vi "Dashboard Main.vi"() -> ()   [LabVIEW 2019]
uses:
  Vision/Vision Mode.ctl
  <vilib>/Utility/miscctls.llb/LVRowAndColumnTypeDef.ctl
  <vilib>/event_ctls.llb/eventvkey.ctl
  <vilib>/Rock Robotics/Network Tables/NT Read Numeric Array.vi
  <vilib>/Rock Robotics/WPI/Dashboard/WPI_DashboardLogging Global.vi
  <vilib>/Rock Robotics/Network Tables/NT Read Boolean.vi
panel:
  in  "Camera Settings Right":T1={"Frame Rate"=30, "Compression"=30, "Size"=1, "DB Camera Config"=FALSE} {"Frame Rate" scale=1.0..30.0; "Compression" scale=100.0..-1.0; "Size" items=["640x480", "320x240", "160x120"]}
  in  "Camera Name Right":string(combo)="No Camera Selection"
  out "Camera Perf":string
  in  "Camera Settings":T1={"Frame Rate"=30, "Compression"=30, "Size"=1, "DB Camera Config"=FALSE} {"Frame Rate" scale=1.0..30.0; "Compression" scale=100.0..-1.0; "Size" items=["640x480", "320x240", "160x120"]}
  in  "TCP":refnum<k5>
  in  "Rec Mode":enum32{"Stop", "Record", "Playback"}(radio)
  out "Robot IP":string
  out "Image Message":string="Timeout in Camera Communications"
  in  "Dashboard Tab":T2(tab)
  in  "Select Auto":string(combo)="Select Autonomous ..."
  out "NT Connection":bool
  out "MotorChart R":cluster{"Numeric":dbl, "Numeric":dbl}(graph)
  out "MotorChart L":cluster{"Numeric":dbl, "Numeric":dbl}(graph)
  out "MotorSliders R":cluster{"MotorSlide1":dbl, "MotorSlide2":dbl} {"MotorSlide2" scale=-1.0..1.0 scale format="%#_2e"; "MotorSlide1" scale=-1.0..1.0 scale format="%#_2e"}
  out "MotorSliders L":cluster{"MotorSlide1":dbl, "MotorSlide2":dbl} {"MotorSlide2" scale=-1.0..1.0 scale format="%#_2e"; "MotorSlide1" scale=-1.0..1.0 scale format="%#_2e"}
  out "Gyro":dbl(knob) scale=0.0..360.0
  out "JS1 Z":dbl(slide) scale=-1.0..1.0 scale format="%#_2e"
  out "JS1 Graph":cluster{"X":dbl, "Y":dbl}[](graph)
  out "JS1 Buttons":T3
  out "JS2 Z":dbl(slide) scale=-1.0..1.0 scale format="%#_2e"
  out "JS2 Graph":cluster{"X":dbl, "Y":dbl}[](graph)
  out "JS2 Buttons":T3
  out "Mode":T4(ring)=enum."Auto Disabled"
  out "Right Camera Perf":cluster{"Bandwidth (Mbps)":dbl, "FPS":dbl}
  out "Camera Image Right":T5(plugin-control)
  in  "DB/String 9":string
  in  "DB/String 8":string
  in  "DB/String 7":string
  in  "DB/String 6":string
  in  "DB/String 5":string
  in  "DB/String 4":string
  in  "DB/String 3":string
  in  "DB/String 2":string
  in  "DB/String 1":string
  in  "DB/String 0":string
  in  "DB/Slider 0":dbl(slide) scale=0.0..5.0
  in  "DB/Slider 1":dbl(slide) scale=0.0..5.0
  in  "DB/Slider 2":dbl(slide) scale=0.0..5.0
  in  "DB/Slider 3":dbl(slide) scale=0.0..5.0
  out "DB/LED 3":bool
  out "DB/LED 2":bool
  out "DB/LED 1":bool
  out "DB/LED 0":bool
  in  "DB/Button 3":bool
  in  "DB/Button 2":bool
  in  "DB/Button 1":bool
  in  "DB/Button 0":bool caption="New Name"
  out "Width":i32
  out "Centroid.x":sgl
  in  "Centerpoint Target":dbl=160.0
  in  "PID gains":T6={"proportional gain (Kc)"=0.01, "integral time (Ti, min)"=0.0, "derivative time (Td, min)"=0.0} {"derivative time (Td, min)" format="%.3f"; "integral time (Ti, min)" format="%.3f"; "proportional gain (Kc)" format="%.3f"}
  in  "Vision Mode":T7
  out "Number of Matches":i32
  in  "Test Slider":dbl(slide) scale=0.0..100.0 scale format="%#_3g"
  in  "On/Off":bool caption="Solenoid"
  in  "Test Name":u16(ring) items=["Select the test to run..."]
  in  "Test Tree":string(tree)
  in  "Motor":cluster{"Value":dbl, "Enable":bool} {"Value" scale=-1.0..1.0 scale format="%#_3g"}
  out "Progress":T8 {"Test Progress" scale=0.0..100.0}
  in  "Rev/Fwd":cluster{"Forward":bool, "Reverse":bool}
  in  "Test Ring":u16(ring) items=["Monochrome", "Color"]
  out "Cmd Status":string
  in  "Execute Command":bool
  in  "Command Params":string[][](table)
  in  "Command Selection":i32(listbox)
  in  "CheckList":i32(listbox)
  out "Tree":string(tree)
  out "Camera Image":T5(plugin-control)
  out "Background":bool
  in  "Camera Name":string(combo)="No Camera Selection"
  # "HW"
  # "HW"
  # "Joysticks"
  # "Drive Motors"
  # "Front"
  # "Right"
  # "Left"
  # "Back"
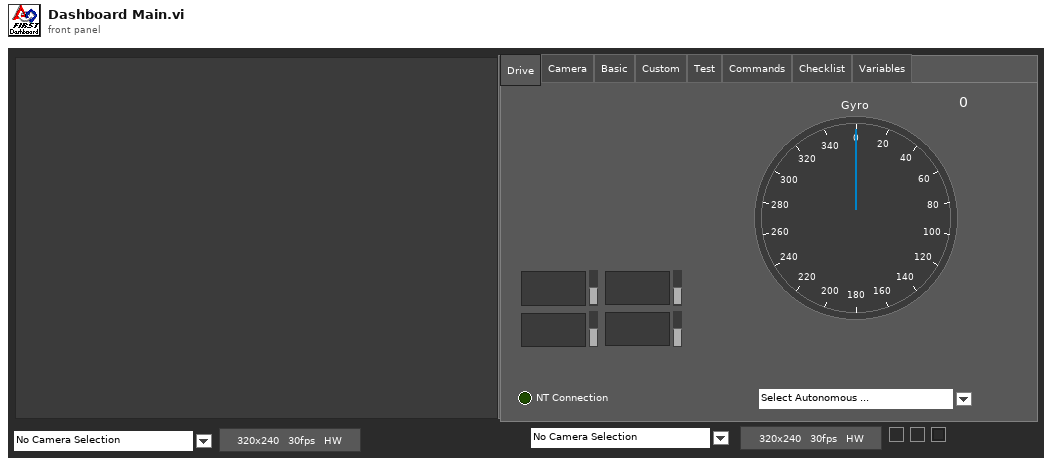
[diagram p1: front panel]
types:
  T1 = cluster{"Frame Rate":i32, "Compression":i32, "Size":u16, "DB Camera Config":bool}
  T2 = enum32{"Drive", "Camera", "Basic", "Custom", "Test", "Commands", "Checklist", "Variables"}
  T3 = cluster{bool, bool, bool, bool, bool, bool, bool, bool, bool, bool, bool, bool}
  T4 = enum8{"Tele-Op Disabled", "Tele-Op Enabled", "Auto Disabled", "Auto Enabled", "Test Disabled", "Test Enabled", "Disconnected", "No Code", "E-Stop"}
  T5 = typedef "IMAQ Image.ctl" = refnum<image>
  T6 = cluster{"proportional gain (Kc)":dbl, "integral time (Ti, min)":dbl, "derivative time (Td, min)":dbl}
  T7 = typedef "Vision Mode.ctl" = enum16{"Rotation", "Translation"}
  T8 = cluster{"Test Progress":u8, "Test Progress Text":string}
  T9 = cluster{"Save Path":path, "Interval (s)":dbl, "Keep":i32}
  T10 = typedef "Image Type" = u32
  T11 = cluster{"IDs":cluster{"RPC field ID":u16, "Unique ID":u16}, "String":string}
  T12 = cluster{"Camera Image":refnum<vi>, "Dashboard Tab":refnum<vi>, "Background":refnum<vi>, "Rec Mode":refnum<vi>, "Test Slider":refnum<vi>, "On/Off ":refnum<vi>, "Test Ring":refnum<vi>, "Rev/Fwd":refnum<vi>, "Test Name":refnum<vi>, "Motor":refnum<vi>, "Progress":refnum<vi>, "CheckList":refnum<vi>, "Tree":refnum<vi>, "Test Tree":refnum<vi>, "Command Params":refnum<vi>, "Command Selection":refnum<vi>, "Execute Command":refnum<vi>, "Cmd Status":refnum<vi>, "Camera Settings":refnum<vi>, "Camera Name":refnum<vi>, "Camera Perf":refnum<vi>, "Camera Settings Right":refnum<vi>, "Camera Name Right":refnum<vi>, "Camera Image Right":refnum<vi>}
  T13 = cluster{"Global Rectangle":i32[], "Contours":cluster{"Contour Type":u32, "ROI Type":u32, "Points":i32[]}[]}
  T14 = cluster{"Camera Name":string, string, "Saved DB Images Info":cluster{"Save Path":path, "Interval (s)":dbl, "Keep":i32}}
  T15 = cluster{"Global Rectangle":cluster{"x1Left":i32, "y1Top":i32, "x2Right":i32, "y2Bottom":i32}, "Centroid":cluster{"x":sgl, "y":sgl}, "Object Size":u32, "Score":dbl}[]
  T16 = cluster{"Error Strings":string, "Disable Counts":cluster{u16, u16}, "Rail Faults":cluster{u16, u16, u16}, "Robot IP":string, "DB Mode":u8, "Event Info":cluster{"Name":string, "Type":u8, "Number":u16, "Replay":u8}}
  T17 = cluster{"Storage":cluster{"Disk Free":u64, "RAM Block":u32, "RAM free":u32}, "CPU Utilization":cluster{"CPU % ISR":sgl, "CPU % Time Crit":sgl, "CPU % Timed Str":sgl, "CPU % High":sgl, "CPU % Above":sgl, "CPU % Normal":sgl, "CPU % Low":sgl}, "CAN":cluster{"% Bus Utilization":sgl, "Bus Off Cnt":u32, "TX_FIFO Full Cnt":u32, "Receive Error Cnt":u8, "Transmit Error Cnt":u8}, "HID":cluster{"HID Outputs":u32, "Rumble Low":u16, "Rumble High":u16}[]}
  T18 = cluster{"Status bits":cluster{"Test Mode":bool, "Autonomous":bool, "Enabled":bool, "Code Start":bool, "Brownout":bool, "Reserved 2":bool, "Reserved 3":bool, "E-Stop":bool}, "Code Trace":cluster{"Disabled":bool, "TeleOp":bool, "Auto":bool, "Test":bool}, "Controller Type":enum16{"unknown", "cRIO", "roboRio"}, "Code?":enum16{"unknown", "noCode", "code"}, "Battery V":dbl}
  T19 = cluster{"Control Bits":cluster{"TestMode":bool, "Autonomous":bool, "Enabled":bool, "FMS Present":bool, bool, bool, bool, "E-Stop":bool}, "Team Station ":u8, "Countdown":sgl, "Joystick Values":cluster{"Axes":dbl[], "Buttons":bool[], "POVs":i16[]}[]}
  T20 = cluster{"Axes":dbl[], "Buttons":bool[], "POVs":i16[]}[]
  T21 = cluster{"Axes":dbl[], "Buttons":bool[], "POVs":i16[]}
  T22 = cluster{"Buttons[0]":bool, "Buttons[1]":bool, "Buttons[2]":bool, "Buttons[3]":bool, "Buttons[4]":bool, "Buttons[5]":bool, "Buttons[6]":bool, "Buttons[7]":bool, "Buttons[8]":bool, "Buttons[9]":bool, "Buttons[10]":bool, "Buttons[11]":bool}
  T23 = cluster{"Camera Name Right":string, string, "Saved DB Images Info":cluster{"Save Path":path, "Interval (s)":dbl, "Keep":i32}}
  T24 = cluster{"Operation":enum16{"Update", "Clear"}, "Color Box":u32}[]
  T25 = typedef "eventvkey.ctl" = enum16{"ASCII", "Enter", "Return", "Shift", "Ctrl", "Alt", "Cmd", "Opt", "Caps", "NumLock", "Clear", "Break", "Up", "Down", "Left", "Right", "Insert", "Delete", "Home", "End", "PageUp", "PageDown", "Escape", "Help", "Pause", "ScrollLock", "F1", "F2", "F3", "F4", "F5", "F6", "F7", "F8", "F9", "F10", "F11", "F12", "F13", "F14", "F15", "F16", "F17", "F18", "F19", "F20", "F21", "F22", "F23", "F24", "Play", "VolumeUp", "VolumeDown", "Mute", "Two Byte Char"}
  T26 = cluster{"Image Size":bool, "Image Type":bool, "Pixel Value":bool, "ROI Information":bool, "Zoom Factor":bool}
  T27 = cluster{"Operation":enum16{"Update", "Clear"}, "Color Box":u32}
  T28 = typedef "LVRowAndColumnTypeDef.ctl" = cluster{"Row":i32, "Column":i32}
  T29 = cluster{"Shift":bool, "Ctrl":bool, "Alt":bool, "Cmd":bool, "Opt":bool}
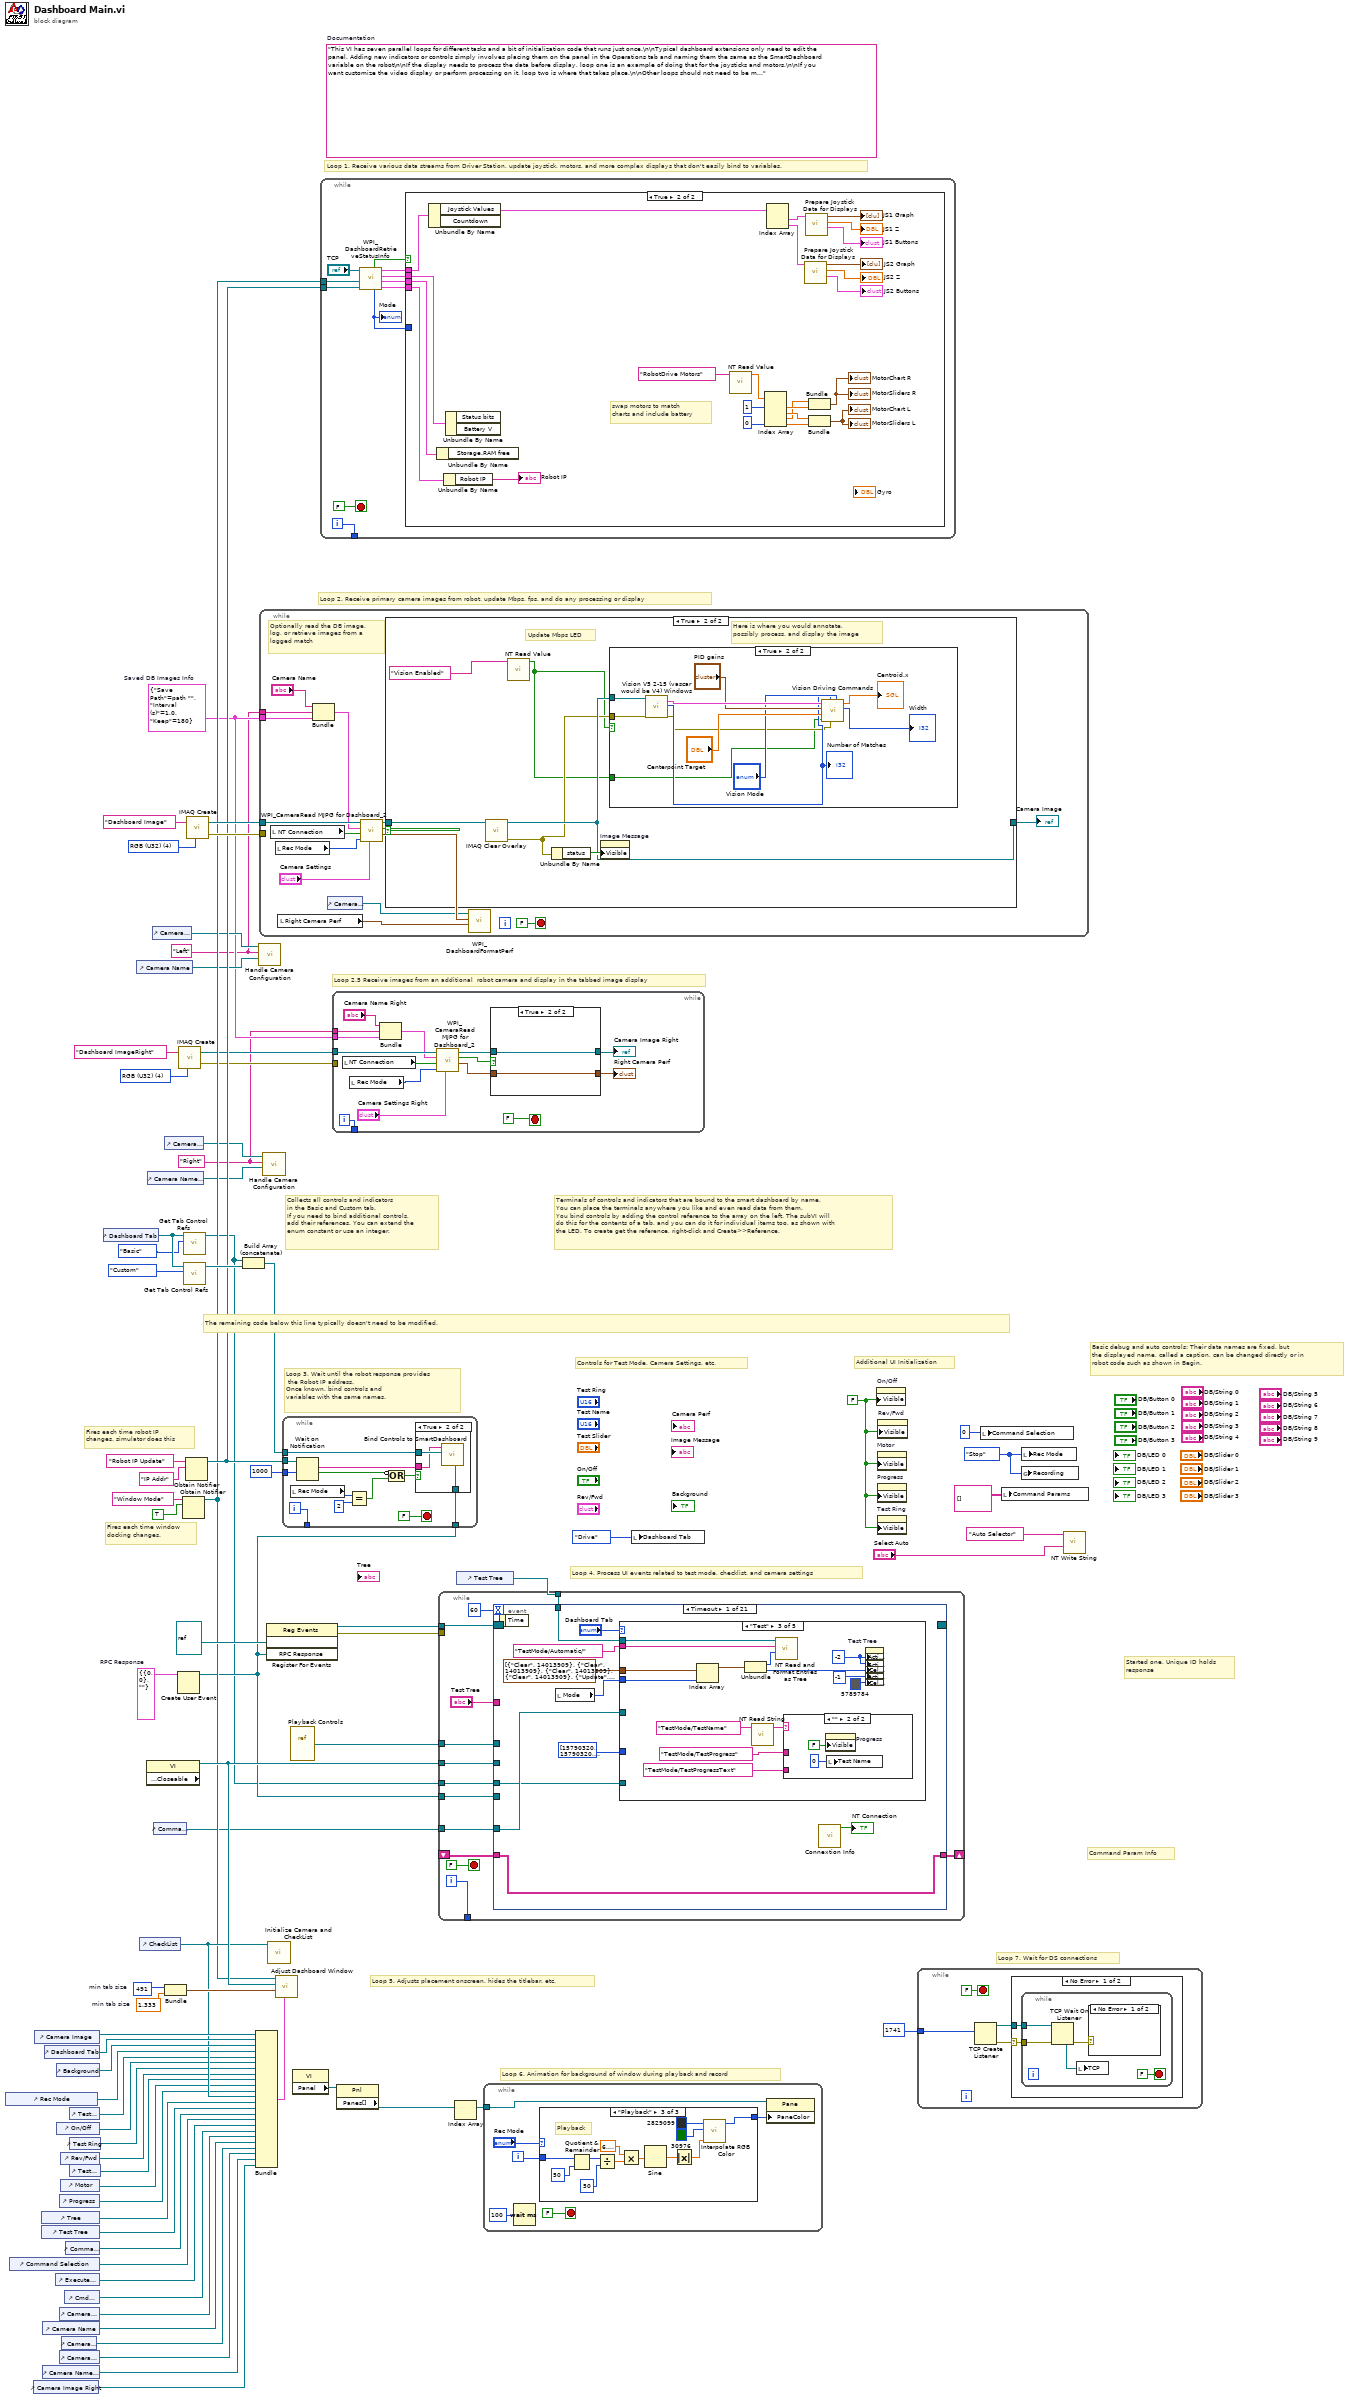
[diagram p0: block diagram]
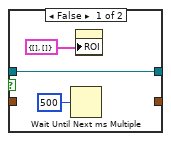
[diagram p2: hidden frame]
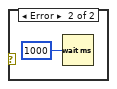
[diagram p3: hidden frame]
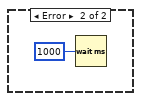
[diagram p4: hidden frame]
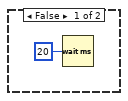
[diagram p5: hidden frame]
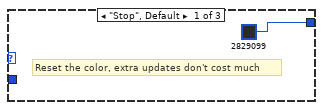
[diagram p6: hidden frame]
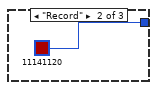
[diagram p7: hidden frame]
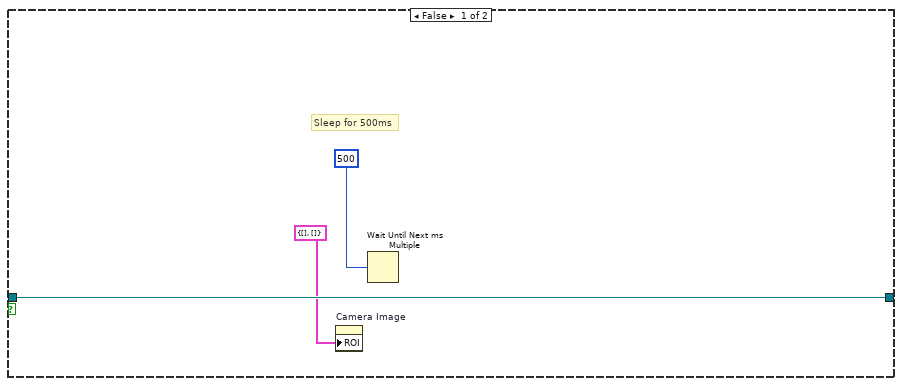
[diagram p9: hidden frame]
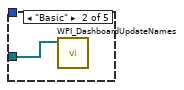
[diagram p12: hidden frame]
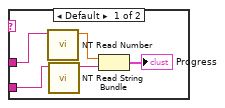
[diagram p13: hidden frame]
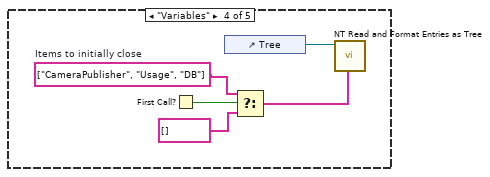
[diagram p14: hidden frame]
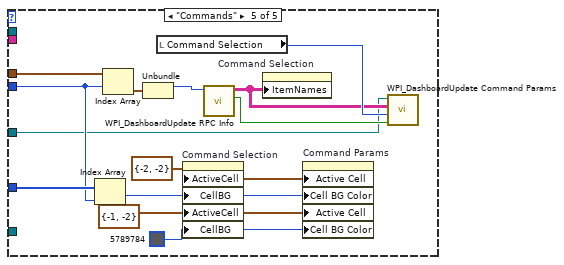
[diagram p15: hidden frame]
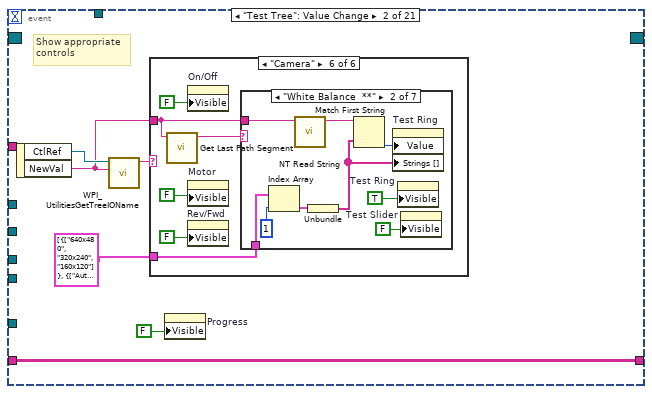
[diagram p16: hidden frame]
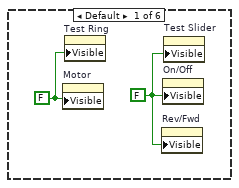
[diagram p17: hidden frame]
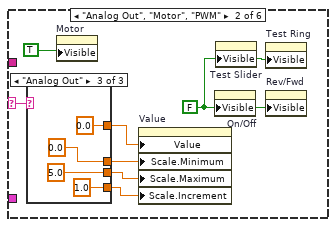
[diagram p18: hidden frame]
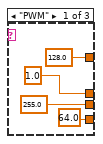
[diagram p19: hidden frame]
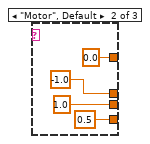
[diagram p20: hidden frame]
diagram:
  w3 = T9 {"Save Path"=path "", "Interval (s)"=1.0, "Keep"=180}  # Saved DB Images Info
  w2 = "Right"
  w1 = "Left"
  w13 = T10 4 items=["Grayscale (U8)", "Grayscale (I16)", "Grayscale (SGL)", "Complex (CSG)", "RGB (U32)", "HSL (U32)", "RGB (U64)"] ("Image Type")
  w29 = T11 {"IDs"={"RPC field ID"=0, "Unique ID"=0}, "String"=""}  # RPC Response
  w52 = 491  # min tab size
  w51 = 1.333  # min tab size
  w59 = enum32{"Stop", "Record", "Playback"}."Stop" ("Rec Mode")
  w36 = FALSE ("Visible")
  (unwired) "This VI has seven parallel loops for different tasks and a bit of initialization code that runs just once.\n\nTypical dashboard extensions only need to edit the panel. Adding new indicators or controls simply involves placing them on the panel in the Operations tab and naming them the same as the SmartDashboard variable on the robot\n\nIf the display needs to process the data before display, loop one is an example of doing that for the joysticks and motors.\n\nIf you want customize the video display or perform processing on it, loop two is where that takes place.\n\nOther loops should not need to be modified. They are pretty standard, and document the task they perform."  # Documentation
  w76 = T10 4 items=["Grayscale (U8)", "Grayscale (I16)", "Grayscale (SGL)", "Complex (CSG)", "RGB (U32)", "HSL (U32)", "RGB (U64)"] ("Image Type")
  # "Loop 2.5 Receive images from an additional  robot camera and display in the tabbed image display"
  # "Command Param Info"
  # "Started one, Unique ID holds\nresponse"
  # "Loop 7. Wait for DS connections"
  # "Basic debug and auto controls: Their data names are fixed, but\nthe displayed name, called a caption, can be changed directly or in\nrobot code such as shown in Begin."
  # "Controls for Test Mode, Camera Settings, etc."
  # "Additional UI Initialization"
  # "Loop 6. Animation for background of window during playback and record"
  # "Fires each time robot IP\nchanges, simulator does this"
  # "Fires each time window\ndocking changes."
  # "Collects all controls and indicators\nin the Basic and Custom tab.\nIf you need to bind additional controls,\nadd their references. You can extend the\nenum constant or use an integer."
  # "The remaining code below this line typically doesn't need to be modified."
  # "Loop 4. Process UI events related to test mode, checklist, and camera settings"
  # "Terminals of controls and indicators that are bound to the smart dashboard by name.\nYou can place the terminals anywhere you like and even read data from them.\nYou bind controls by adding the control reference to the array on the left. The subVI will\ndo this for the contents of a tab, and you can do it for individual items too, as shown with\nthe LED. To create get the reference, right-click and Create>>Reference."
  # "Loop 3. Wait until the robot response provides\n the Robot IP address.\nOnce known, bind controls and\nvariables with the same names."
  # "Loop 5. Adjusts placement onscreen, hides the titlebar, etc."
  # "Loop 1. Receive various data streams from Driver Station, update joystick, motors, and more complex displays that don't easily bind to variables."
  # "Loop 2. Receive primary camera images from robot, update Mbps, fps, and do any processing or display"
  n1 = control-ref of="Rec Mode"() -> (w42:refnum<vi>)
  n2 = control-ref of="Command Selection"() -> (w28:refnum<vi>)
  n3 = control-ref of="Camera Image Right"() -> (w6:refnum<vi>)
  n4 = control-ref of="Camera Image"() -> (w54:refnum<vi>)
  n5 = control-ref of="Tree"() -> (w46:refnum<vi>)
  n6 = control-ref of="Test Tree"() -> (w45:refnum<vi>)
  n7 = control-ref of="Camera Name"() -> (w19:refnum<vi>)
  n8 = control-ref of="Camera Name Right"() -> (w7:refnum<vi>)
  n9 = control-ref of="Dashboard Tab"() -> (w53:refnum<vi>)
  n10 = control-ref of="Execute Command"() -> (w30:refnum<vi>)
  n11 = control-ref of="Background"() -> (w49:refnum<vi>)
  n12 = control-ref of="On/Off"() -> (w40:refnum<vi>)
  n13 = control-ref of="Progress"() -> (w37:refnum<vi>)
  n14 = control-ref of="Camera Settings"() -> (w20:refnum<vi>)
  n15 = control-ref of="Camera Settings Right"() -> (w8:refnum<vi>)
  n16 = control-ref of="Rev/Fwd"() -> (w38:refnum<vi>)
  n17 = control-ref of="Motor"() -> (w43:refnum<vi>)
  n18 = control-ref of="Camera Perf"() -> (w18:refnum<vi>)
  n19 = control-ref of="Cmd Status"() -> (w24:refnum<vi>)
  n20 = control-ref of="Command Params"() -> (w31:refnum<vi>)
  n21 = control-ref of="Test Slider"() -> (w41:refnum<vi>)
  n22 = control-ref of="Test Ring"() -> (w39:refnum<vi>)
  n23 = control-ref of="Test Name"() -> (w44:refnum<vi>)
  n24 = control-ref of="Dashboard Tab"() -> (w57:refnum<vi>)
  n25 = control-ref of="Camera Name"() -> (w21:refnum<vi>)
  n26 = control-ref of="CheckList"() -> (w47:refnum<vi>)
  n27 = property class="VI" props=["Front Panel.Closeable"]() -> (reference out=w58:refnum<vi>)  [unwired: 2 in, 2 out]
  n28 = control-ref of="Camera Name Right"() -> (w9:refnum<vi>)
  n29 = control-ref of="Camera Settings"() -> (w22:refnum<vi>)
  n30 = control-ref of="Command Params"() -> (w23:refnum<vi>)
  n31 = control-ref of="Camera Settings Right"() -> (w10:refnum<vi>)
  n32 = Bundle("min tab size"=w52, "min tab size"=w51) -> (w50:cluster{"min tab size":i32, "min tab size":dbl})  [unwired: 1 in]
  n33 = Create User Event(user event datatype=w29) -> (user event=w25:refnum<user-event>)  [unwired: 1 in, 1 out]
  n34 = call "IMAQ Create"("Image Name"="Dashboard ImageRight", "Image Type"=w13) -> ("New Image"=w12:T5, "error out"=w11:errorcluster)  [unwired: 2 in, 1 out]
  n35 = Obtain Notifier(name (unnamed)="Window Mode", notification data type=TRUE) -> (notifier out=w34:refnum<notifier>)  [unwired: 2 in, 2 out]
  n36 = call <vilib>:"Get Tab Control Refs.vi"("Page Index"=T2."Basic" ("Dashboard Tab"), "TabControl in"=w57) -> ("ControlsOnPage"=w17:refnum<vi>[])  [unwired: 9 in]
  n37 = call <vilib>:"Get Tab Control Refs.vi"("Page Index"=T2."Custom" ("Dashboard Tab"), "TabControl in"=w57) -> ("ControlsOnPage"=w56:refnum<vi>[])  [unwired: 9 in]
  n38 = Obtain Notifier(name (unnamed)="Robot IP Update", notification data type="IP Addr" ("name (unnamed)")) -> (notifier out=w35:refnum<notifier>)  [unwired: 2 in, 2 out]
  n39 = call "IMAQ Create"("Image Name"="Dashboard Image", "Image Type"=w76) -> ("New Image"=w74:T5, "error out"=w73:errorcluster)  [unwired: 2 in, 1 out]
  n40 = Build Array (concatenate)(w17, w56) -> (w55:refnum<vi>[])
  n41 = Bundle("Camera Image"=w54, "Dashboard Tab"=w53, "Background"=w49, "Rec Mode"=w42, "Test Slider"=w41, "On/Off"=w40, "Test Ring"=w39, "Rev/Fwd"=w38, "Test Name"=w44, "Motor"=w43, "Progress"=w37, "CheckList"=w47, "Tree"=w46, "Test Tree"=w45, "Command Params"=w31, "Command Selection"=w28, "Execute Command"=w30, "Cmd Status"=w24, "Camera Settings"=w20, "Camera Name"=w19, "Camera Perf"=w18, "Camera Settings Right"=w8, "Camera Name Right"=w7, "Camera Image Right"=w6) -> (w48:T12)  [unwired: 1 in]
  n42 = call "Handle Camera Configuration.vi"("CameraNameRef"=w21, "Display Name"=w1, "ClusterRef"=w22) -> ()  [unwired: 9 in]
  n43 = while {
    tunnel: w74 -> [w90]
    tunnel: w73 -> [_]
    tunnel: w3 -> [w83]
    tunnel: w1 -> [w80]
    stop <- FALSE stop-if-true
    # "Optionally read the DB image,\nlog, or retrieve images from a\nlogged match"
    n44 = local read "NT Connection"() -> (w84:bool)
    n45 = local read "Rec Mode"() -> (w87:enum32{"Stop", "Record", "Playback"})
    n46 = local read "Right Camera Perf"() -> (w78:cluster{"Bandwidth (Mbps)":dbl, "FPS":dbl})
    n47 = Bundle("Camera Name"="Camera Name", w80, "Saved DB Images Info"=w83) -> (w82:T14)  [unwired: 1 in]
    n48 = control-ref of="Camera Perf"() -> (w77:refnum<vi>)
    n49 = call <vilib>:"WPI_CameraRead MJPG for Dashboard_2.vi"("Camera Settings"="Camera Settings", "Rec Mode"=w87, "NT Connection"=w84, "Capture Info"=w82, "Image in"=w90) -> ("perf info"=w79:cluster{"Bandwidth (Mbps)":dbl, "fps":dbl}, "Active"=w88:bool, "Image\\ out"=w89:T5)  [unwired: 4 in]
    n50 = case shown="True" w88 {
      tunnel: w89 -> [w93 w99]
      tunnel: [w93 w98] -> w85
      frame False {
        # "Sleep for 500ms"
        n51 = property on="Camera Image" class="ImageControl"("ROI"=T13 {"Global Rectangle"=[], "Contours"=[]}) -> ()  [unwired: 2 in, 2 out]
        n52 = Wait Until Next ms Multiple(millisecond multiple=u32 500) -> ()  [unwired: 1 out]
      }
      frame True {
        # "Here is where you would annotate,\npossibly process, and display the image"
        # "Update Mbps LED"
        n53 = call "IMAQ Clear Overlay"("Image"=w99) -> ("error out"=w97:errorcluster, "Image Out"=w98:T5)  [unwired: 2 in, 7 out]
        n54 = call-poly <vilib>:"NT Read Value.vi"("Name"="Vision Enabled") -> ("Boolean"=w95:bool)  [unwired: 9 in, 1 out]
        n55 = Unbundle By Name(w97) -> ("status"=w100:bool)
        n56 = property on="Image Message" class="Str"("Visible"=w100) -> ()  [unwired: 2 in, 2 out]
        n57 = case shown="True" w95 {
          tunnel: w98 -> [_ w111]
          tunnel: w97 -> [_ w109]
          tunnel: w95 -> [_ w101]
          frame False {
          }
          frame True {
            n58 = call "Vision V5 2-15 (vascar would be V4) Windows.vi"("Image in"=w111, "error in"=w109) -> ("Shape Report (calibrated)"=w110:T15, "Number of Matches"=w103:i32, "error out"=w102:errorcluster)  [unwired: 14 in, 1 out]
            "Number of Matches" <- w103
            n59 = call "Vision Driving Commands.vi"("Vision Mode"="Vision Mode", "error in (no error)"=w102, "Number of Matches"=w103, "Vision Enabled"=w101, "Centerpoint Target"="Centerpoint Target", "PID gains"="PID gains", "Shape Report (calibrated)"=w110) -> ("Width"=→"Width":i32, "Centroid.x"=→"Centroid.x":sgl)  [unwired: 3 in]
          }
        }
      }
    }
    "Camera Image" <- w85
    n60 = call <vilib>:"WPI_DashboardFormatPerf.vi"("Right Camera Perf"=w78, "Performance"=w79, "String in"=w77) -> ()  [unwired: 9 in]
  }
  n61 = call "Handle Camera Configuration.vi"("CameraNameRef"=w9, "Display Name"=w2, "ClusterRef"=w10) -> ()  [unwired: 9 in]
  n62 = register-events(refnum<vi> refnum, w25) -> (reference out=w63:refnum<event-registration>, error out=w62:errorcluster)  [unwired: 2 in]
  n63 = call "Initialize Camera and CheckList.vi"("ListBox in"=w47) -> ()  [unwired: 11 in]
  n64 = call "Adjust Dashboard Window.vi"("Sizing Refnums"=w48, "Size Constraints"=w50, "VI"=w58, "WIn Mode"=w34) -> ()  [unwired: 8 in]
  n65 = while {
    tunnel: w55 -> [w123]
    tunnel: w35 -> [w121]
    tunnel: [w119] -> _
    tunnel: u32 1000 ("milliseconds to wait") -> [w118]
    tunnel: w25 -> [w112]
    i -> [w119]
    stop <- FALSE stop-if-true
    n66 = local read "Rec Mode"() -> (w114:enum32{"Stop", "Record", "Playback"})
    n67 = Wait on Notification(notifier=w121, timeout in ms (-1)=w118) -> (notification=w120:string, timed out?=w116:bool)  [unwired: 2 in, 2 out]
    n68 = Equal?(x=w114, y=u16 2 ("Rec Mode")) -> (x = y?=w115:bool)
    n69 = Compound Arithmetic op=OR(invert w116, w115) -> (w117:bool)
    n70 = case shown="True" w117 {
      tunnel: w123 -> [_ w126]
      tunnel: w120 -> [_ w125]
      tunnel: w112 -> [_ w124]
      frame False {
      }
      frame True {
        n71 = call <vilib>:"Bind Controls to SmartDashboard.vi"("RPC ref"=w124, "Bound Control Refs"=w126, "Server IP Address"=w125) -> ()  [unwired: 9 in]
      }
    }
  }
  n72 = vi-ref "Playback Controls.vi"() -> (w64:refnum<vi>)
  n73 = property class="VI"() -> ("Panel"=w66:refnum<vi>)  [unwired: 2 in, 2 out]
  n74 = while {
    tunnel: [w136] -> _
    tunnel: w35 -> [w130]
    tunnel: w34 -> [w127]
    i -> [w136]
    stop <- FALSE stop-if-true
    n75 = call <vilib>:"WPI_DashboardRetrieveStatusInfo.vi"("Binding Refnum"=w130, "Window Mode Notifier"=w127, "TCP Cnx"="TCP") -> ("Power and Errors"=w131:T16, "Robot Metrics"=w134:T17, "Status Info"=w135:T18, "Control Info"=w132:T19, "Robot Mode"=w129:T4, "Process?"=w133:bool)  [unwired: 3 in]
    "Mode" <- w129
    n76 = case shown="True" w133 {
      tunnel: w135 -> [_ w162]
      tunnel: w134 -> [_ w161]
      tunnel: w132 -> [_ w160]
      tunnel: w131 -> [_ w159]
      tunnel: w129 -> [_ _]
      frame False {
        n77 = Wait (ms)(milliseconds to wait=u32 20) -> ()  [unwired: 1 out]
      }
      frame True {
        # "swap motors to match\ncharts and include battery"
        n78 = Unbundle By Name(w160) -> ("Joystick Values"=w150:T20)  [unwired: 1 out]
        n79 = Unbundle By Name(w161) -> ()  [unwired: 1 out]
        n80 = Unbundle By Name(w159) -> ("Robot IP"=→"Robot IP":string)
        n81 = Unbundle By Name(w162) -> ()  [unwired: 2 out]
        n82 = call-poly <vilib>:"NT Read Value.vi"("Name"="RobotDrive Motors") -> ("Numeric Array"=w140:dbl[])  [unwired: 9 in, 1 out]
        n83 = Index Array(array=w140, index #1=1, index #4=0) -> (element #1=w154:dbl, element #2=w155:dbl, element #3=w153:dbl, element #4=w158:dbl)  [unwired: 2 in]
        n84 = Index Array(array=w150) -> (element #1=w149:T21, element #2=w145:T21)  [unwired: 2 in]
        n85 = call "Prepare Joystick Data for Displays.vi"("Joystick Values"=w145) -> ("Buttons"=→"JS2 Buttons":T22, "Z Axis"=→"JS2 Z":dbl, "Cartesian Data"=→"JS2 Graph":cluster{"X axis":dbl, "X axis":dbl}[])  [unwired: 8 in]
        n86 = call "Prepare Joystick Data for Displays.vi"("Joystick Values"=w149) -> ("Buttons"=→"JS1 Buttons":T22, "Z Axis"=→"JS1 Z":dbl, "Cartesian Data"=→"JS1 Graph":cluster{"X axis":dbl, "X axis":dbl}[])  [unwired: 8 in]
        n87 = Bundle("Numeric"=w153, "Numeric"=w154) -> (→"MotorChart R" →"MotorSliders R":cluster{"Numeric":dbl, "Numeric":dbl})  [unwired: 1 in]
        n88 = Bundle("Numeric"=w155, "Numeric"=w158) -> (→"MotorChart L" →"MotorSliders L":cluster{"Numeric":dbl, "Numeric":dbl})  [unwired: 1 in]
      }
    }
  }
  n89 = while {
    tunnel: w12 -> [w177]
    tunnel: w11 -> [_]
    tunnel: [w172] -> _
    tunnel: w3 -> [w168]
    tunnel: w2 -> [w165]
    i -> [w172]
    stop <- FALSE stop-if-true
    n90 = local read "NT Connection"() -> (w169:bool)
    n91 = local read "Rec Mode"() -> (w176:enum32{"Stop", "Record", "Playback"})
    n92 = Bundle("Camera Name Right"="Camera Name Right", w165, "Saved DB Images Info"=w168) -> (w167:T23)  [unwired: 1 in]
    n93 = call <vilib>:"WPI_CameraRead MJPG for Dashboard_2.vi"("Camera Settings"="Camera Settings Right", "Rec Mode"=w176, "NT Connection"=w169, "Capture Info"=w167, "Image in"=w177) -> ("perf info"=w163:cluster{"Bandwidth (Mbps)":dbl, "fps":dbl}, "Active"=w171:bool, "Image\\ out"=w174:T5)  [unwired: 4 in]
    n94 = case shown="True" w171 {
      tunnel: w174 -> [w179 w182]
      tunnel: [w179 w182] -> w170
      tunnel: [_ w181] -> w164
      tunnel: w163 -> [_ w181]
      frame False {
        n95 = Wait Until Next ms Multiple(millisecond multiple=u32 500) -> ()  [unwired: 1 out]
        n96 = property on="Camera Image Right" class="ImageControl"("ROI"=T13 {"Global Rectangle"=[], "Contours"=[]}) -> ()  [unwired: 2 in, 2 out]
      }
      frame True {
      }
    }
    "Camera Image Right" <- w170
    "Right Camera Perf" <- w164
  }
  n97 = property class="Pnl"(reference=w66) -> ("Panes[]"=w67:refnum<vi>[])  [unwired: 1 in, 2 out]
  n98 = Index Array(array=w67) -> (element=w65:refnum<vi>)  [unwired: 1 in]
  n99 = control-ref of="Test Tree"() -> (w68:refnum<vi>)
  n100 = while {
    tunnel: [w192] -> _
    tunnel: w68 -> [w191]
    tunnel: w64 -> [w190]
    tunnel: w63 -> [w189]
    tunnel: w62 -> [_]
    tunnel: w58 -> [w188]
    tunnel: w25 -> [w187]
    tunnel: w23 -> [w186]
    shift-right: [w185] -> _
    shift-left: _ -> [w184]
    tunnel: w17 -> [w183]
    i -> [w192]
    stop <- FALSE stop-if-true
    n101 = event shown="[0] Timeout" {
      selector: w189 -> [_ _ _ _ _ _ _ _ _ _ _ _ _ _ _ _ _ _ _ _ _]
      dyn-events: [_ _ _ _ _ _ _ _ _ _ _ _ _ _ _ _ w452 _ _ _ _] -> _
      timeout: u32 60 ("milliseconds to wait") -> [_ _ _ _ _ _ _ _ _ _ _ _ _ _ _ _ _ _ _ _ _]
      tunnel: w191 -> [w204 _ _ _ _ _ _ _ _ _ _ _ _ _ _ _ _ _ _ _ _]
      tunnel: "Test Tree" -> [_ _ _ _ _ _ _ _ _ _ _ w419 w427 w429 w433 w441 _ _ _ _ _]
      tunnel: w190 -> [_ _ _ _ _ _ _ _ _ _ _ _ _ _ _ _ w454 _ w472 _ _]
      tunnel: w188 -> [_ _ _ _ _ _ _ _ _ _ _ _ _ _ _ _ w450 _ _ _ _]
      tunnel: w187 -> [_ _ _ _ _ _ _ _ _ _ _ _ _ _ _ _ w448 _ _ _ _]
      tunnel: w186 -> [w199 _ _ _ _ _ w370 _ _ _ _ _ _ _ _ _ _ _ _ _ _]
      tunnel: [w198 w247 w349 w354 w363 w367 w368 w377 w387 w394 w406 w418 w425 w428 w432 w440 w447 w467 w469 w473 w486] -> w185
      tunnel: w184 -> [w198 w247 w349 w354 w363 w367 w368 _ _ w394 w406 w418 w425 w428 w432 w440 w447 w467 w469 w473 w486]
      tunnel: w183 -> [w196 _ _ _ _ _ _ _ _ _ _ _ _ _ _ _ _ _ _ _ _]
      event Timeout {
        n102 = event-data() -> ()  [unwired: 1 in, 1 out]
        n103 = local read "Mode"() -> (w201:T4)
        n104 = case shown="\"Test\"" "Dashboard Tab" {
          tunnel: w204 -> [_ _ w220 _ _]
          tunnel: "TestMode/Automatic/" ("Name Pattern") -> [_ _ w219 _ _]
          tunnel: T24 [{"Operation"=enum."Clear", "Color Box"=14013909}, {"Operation"=enum."Clear", "Color Box"=14013909}, {"Operation"=enum."Clear", "Color Box"=14013909}, {"Operation"=enum."Clear", "Color Box"=14013909}, {"Operation"=enum."Update", "Color Box"=14013909}, {"Operation"=enum."Update", "Color Box"=16777215}, {"Operation"=enum."Clear", "Color Box"=14013909}, {"Operation"=enum."Clear", "Color Box"=14013909}, {"Operation"=enum."Clear", "Color Box"=14013909}] -> [_ _ w212 _ w240]
          tunnel: w201 -> [_ _ w211 _ w239]
          tunnel: u32[] [15790320, 15790320, 15790320, 15790320, 16777215, 16777215, 15790320, 15790320, 15790320] -> [_ _ _ _ w245]
          tunnel: w199 -> [_ _ _ _ w233]
          tunnel: w196 -> [_ w206 _ _ _]
          frame "Custom", Default {
          }
          frame "Basic" {
            n105 = call <vilib>:"WPI_DashboardUpdateNames.vi"("Controls on Tab"=w206) -> ()  [unwired: 11 in]
          }
          frame "Test" {
            w218 = -2 ("Active Item:Row Number")
            n106 = Index Array(array=w212, index=w211) -> (element=w213:T27)
            n107 = Unbundle(w213) -> ("Operation"=w214:enum16{"Update", "Clear"}, "Color Box"=w215:u32)
            n108 = call <vilib>:"NT Read String.vi"("Name"="TestMode/TestName") -> ("String"=w209:string)  [unwired: 9 in, 1 out]
            n109 = call <vilib>:"NT Read and Format Entries as Tree.vi"("Operation"=w214, "Name Pattern"=w219, "Tree Refnum"=w220) -> ()  [unwired: 7 in, 2 out]
            n110 = case shown="\"\"" w209 {
              tunnel: "TestMode/TestProgress" ("Name") -> [w222 _]
              tunnel: "TestMode/TestProgressText" ("Name") -> [w221 _]
              frame Default {
                n111 = call <vilib>:"NT Read Number.vi"("Name"=w222) -> ("Numeric"=w223:dbl)  [unwired: 9 in, 1 out]
                n112 = call <vilib>:"NT Read String.vi"("Name"=w221) -> ("String"=w224:string)  [unwired: 9 in, 1 out]
                n113 = Bundle("Numeric"=w223, "String"=w224) -> (→"Progress":cluster{"Numeric":dbl, "String":string})  [unwired: 1 in]
              }
              frame "" {
                n114 = property on="Progress" class="Clust (strict)"("Visible"=FALSE) -> ()  [unwired: 2 in, 2 out]
                n115 = local write "Test Name"(u16 0) -> ()
              }
            }
            n116 = property on="Test Tree" class="Tree (strict)"("Active Item Row Number"=w218, "ActiveColNum"=w218, "CellBG"=w215, "Active Item Row Number"=-1 ("Active Item:Row Number"), "CellBG"=u32 5789784 ("Color Box")) -> ()  [unwired: 2 in, 2 out]
          }
          frame "Variables" {
            w230 = string[] ["CameraPublisher", "Usage", "DB"]  # Items to initially close
            n117 = First Call?() -> (First Call?: T/F=w231:bool)
            n118 = control-ref of="Tree"() -> (w232:refnum<vi>)
            n119 = Select(t=w230, s=w231, f=string[] []) -> (s? t:f=w228:string[])
            n120 = call <vilib>:"NT Read and Format Entries as Tree.vi"("Tags to  Close"=w228, "Tree Refnum"=w232) -> ()  [unwired: 8 in, 2 out]
          }
          frame "Commands" {
            w241 = u32 5789784 ("Color Box")
            w242 = T28 {"Row"=-1, "Column"=-2} ("Active Cell:Active Cell")
            w244 = T28 {"Row"=-2, "Column"=-2} ("Active Cell:Active Cell")
            n121 = Index Array(array=w245, index=w239) -> (element=w243:u32)
            n122 = Index Array(array=w240, index=w239) -> (element=w238:T27)
            n123 = Unbundle(w238) -> ("Operation"=w237:enum16{"Update", "Clear"})  [unwired: 1 out]
            n124 = local read "Command Selection"() -> (w236:i32)
            n125 = property on="Command Selection" class="MCListbox (strict)"("ActiveCell"=w244, "CellBG"=w243, "ActiveCell"=w242, "CellBG"=w241) -> ()  [unwired: 2 in, 2 out]
            n126 = call <vilib>:"WPI_DashboardUpdate RPC Info.vi"("Operation"=w237) -> ("update"=w235:bool, "commands"=w234:string[][])  [unwired: 9 in]
            n127 = property on="Command Selection" class="MCListbox (strict)"("ItemNames"=w234) -> ()  [unwired: 2 in, 2 out]
            n128 = property on="Command Params" class="Tbl (strict)"("Active Cell"=w244, "Cell BG Color"=w243, "Active Cell"=w242, "Cell BG Color"=w241) -> ()  [unwired: 2 in, 2 out]
            n129 = call <vilib>:"WPI_DashboardUpdate Command Params.vi"("Update"=w235, "NewVal"=w236, "Commands"=w234, "Param Tbl"=w233) -> ()  [unwired: 7 in, 1 out]
          }
        }
        n130 = call <vilib>:"Connextion Info.vi"() -> ("Connected"=→"NT Connection":bool)  [unwired: 10 in, 1 out]
      }
      event "Test Tree": Value Change {
        # "Show appropriate\ncontrols"
        n131 = event-data() -> ("CtlRef"=w250:refnum<vi>, "NewVal"=w248:string)  [unwired: 1 in]
        n132 = call <vilib>:"WPI_UtilitiesGetTreeIOName.vi"("NewVal"=w248, "TreeControl in"=w250) -> ("I/O Name"=w251:string)  [unwired: 9 in]
        n133 = case shown="\"Camera\"" w251 {
          selector: w251 -> [_ w258 _ w280 w289 _]
          tunnel: w248 -> [_ _ w277 w279 _ w296]
          tunnel: cluster{string[]}[] [{["640x480", "320x240", "160x120"]}, {["Auto", "Fixed indoor", "Fixed outdoor 1", "Fixed outdoor 2", "Fixed fluorescent 1", "Fixed fluorescent 2", "Hold current"]}, {["Auto", "Flicker-free 50 Hz", "Flicker-free 60 Hz", "Hold current"]}, {["None", "Prioritize frame rate", "Prioritize image quality"]}, {["Monochrome", "Color"]}] -> [_ _ _ _ _ w295]
          frame Default {
            w253 = FALSE ("Visible")
            w252 = FALSE ("Visible")
            n134 = property on="Motor" class="Clust (strict)"("Visible"=w252) -> ()  [unwired: 2 in, 2 out]
            n135 = property on="Test Ring" class="Ring (strict)"("Visible"=w252) -> ()  [unwired: 2 in, 2 out]
            n136 = property on="Rev/Fwd" class="Clust (strict)"("Visible"=w253) -> ()  [unwired: 2 in, 2 out]
            n137 = property on="On/Off" class="Bool (strict)"("Visible"=w253) -> ()  [unwired: 2 in, 2 out]
            n138 = property on="Test Slider" class="Slide (strict)"("Visible"=w253) -> ()  [unwired: 2 in, 2 out]
          }
          frame "Analog Out", "Motor", "PWM" {
            w259 = FALSE ("Visible")
            n139 = case shown="\"Analog Out\"" w258 {
              tunnel: [1.0 ("Value") -1.0 ("Value") 0.0 ("Value")] -> w257
              tunnel: [255.0 ("Value") 1.0 ("Value") 5.0 ("Value")] -> w256
              tunnel: [128.0 ("Value") 0.0 ("Value") 0.0 ("Value")] -> w255
              tunnel: [64.0 ("Value") 0.5 ("Value") 1.0 ("Value")] -> w254
              frame "PWM" {
              }
              frame "Motor", Default {
              }
              frame "Analog Out" {
              }
            }
            n140 = property on="Motor" class="Clust (strict)"("Visible"=TRUE) -> ()  [unwired: 2 in, 2 out]
            n141 = property on="Value" class="Slide (strict)"("Value"=w255, "Scale.Minimum"=w257, "Scale.Maximum"=w256, "Scale.Increment"=w254) -> ()  [unwired: 2 in, 2 out]
            n142 = property on="On/Off" class="Bool (strict)"("Visible"=w259) -> ()  [unwired: 2 in, 2 out]
            n143 = property on="Test Slider" class="Slide (strict)"("Visible"=w259) -> ()  [unwired: 2 in, 2 out]
            n144 = property on="Test Ring" class="Ring (strict)"("Visible"=w259) -> ()  [unwired: 2 in, 2 out]
            n145 = property on="Rev/Fwd" class="Clust (strict)"("Visible"=w259) -> ()  [unwired: 2 in, 2 out]
          }
          frame "Servo" {
            w275 = FALSE ("Visible")
            n146 = call <vilib>:"NT Read Number.vi"("Name"=w277) -> ("Numeric"=w276:dbl)  [unwired: 9 in, 1 out]
            n147 = property on="Test Slider" class="Slide (strict)"("Visible"=TRUE, "Scale.Maximum"=170.0 ("Scale.Range:Maximum")) -> ()  [unwired: 2 in, 2 out]
            n148 = local write "Test Slider"(w276) -> ()
            n149 = property on="Motor" class="Clust (strict)"("Visible"=w275) -> ()  [unwired: 2 in, 2 out]
            n150 = property on="Rev/Fwd" class="Clust (strict)"("Visible"=w275) -> ()  [unwired: 2 in, 2 out]
            n151 = property on="On/Off" class="Bool (strict)"("Visible"=w275) -> ()  [unwired: 2 in, 2 out]
            n152 = property on="Test Ring" class="Ring (strict)"("Visible"=w275) -> ()  [unwired: 2 in, 2 out]
          }
          frame "Relay", "Solenoid" {
            w278 = FALSE ("Visible")
            n153 = property on="Motor" class="Clust (strict)"("Visible"=w278) -> ()  [unwired: 2 in, 2 out]
            n154 = property on="Test Slider" class="Slide (strict)"("Visible"=w278) -> ()  [unwired: 2 in, 2 out]
            n155 = Search and Replace String(input string=w279, search string="/Value  **", replace string="/Direction") -> (result string=w285:string)  [unwired: 5 in, 3 out]
            n156 = property on="Test Ring" class="Ring (strict)"("Visible"=w278) -> ()  [unwired: 2 in, 2 out]
            n157 = call <vilib>:"NT Read String.vi"("Name"=w285) -> ("String"=w283:string)  [unwired: 9 in, 1 out]
            n158 = Equal?(x="Both directions", y=w283) -> (x = y?=w281:bool)
            n159 = Not(x=w281) -> (.not. x?=w282:bool)
            n160 = property on="Rev/Fwd" class="Clust (strict)"("Visible"=w281) -> ()  [unwired: 2 in, 2 out]
            n161 = property on="On/Off" class="Bool (strict)"("Visible"=w282, "Caption.Text"=w280) -> ()  [unwired: 2 in, 2 out]
          }
          frame "Compressor", "Digital Out" {
            w288 = FALSE ("Visible")
            # "Get direction and finish"
            n162 = property on="Motor" class="Clust (strict)"("Visible"=w288) -> ()  [unwired: 2 in, 2 out]
            n163 = property on="Test Slider" class="Slide (strict)"("Visible"=w288) -> ()  [unwired: 2 in, 2 out]
            n164 = property on="Test Ring" class="Ring (strict)"("Visible"=w288) -> ()  [unwired: 2 in, 2 out]
            n165 = property on="On/Off" class="Bool (strict)"("Visible"=TRUE, "Caption.Text"=w289) -> ()  [unwired: 2 in, 2 out]
            n166 = property on="Rev/Fwd" class="Clust (strict)"("Visible"=FALSE) -> ()  [unwired: 2 in, 2 out]
          }
          frame "Camera" {
            n167 = call <vilib>:"Get Last Path Segment.vi"("String in"=w296) -> ("String out"=w297:string)  [unwired: 10 in]
            n168 = property on="On/Off" class="Bool (strict)"("Visible"=FALSE) -> ()  [unwired: 2 in, 2 out]
            n169 = property on="Motor" class="Clust (strict)"("Visible"=FALSE) -> ()  [unwired: 2 in, 2 out]
            n170 = property on="Rev/Fwd" class="Clust (strict)"("Visible"=FALSE) -> ()  [unwired: 2 in, 2 out]
            n171 = case shown="\"White Balance  **\"" w297 {
              tunnel: w296 -> [w303 w312 w321 w330 w339 _ w345]
              tunnel: w295 -> [w301 w309 w318 w327 w336 _ _]
              frame "Size  **" {
                n172 = Index Array(array=w301) -> (element=w300:cluster{string[]})  [unwired: 1 in]
                n173 = call <vilib>:"NT Read String.vi"("Name"=w303) -> ("String"=w302:string)  [unwired: 9 in, 1 out]
                n174 = Unbundle(w300) -> (w298:string[])
                n175 = Match First String(2:w298, 3:w302) -> (0:w299:i32)  [unwired: 1 out]
                n176 = property on="Test Ring" class="Ring (strict)"("Value"=w299, "Strings []"=w298) -> ()  [unwired: 2 in, 2 out]
                n177 = property on="Test Ring" class="Ring (strict)"("Visible"=TRUE) -> ()  [unwired: 2 in, 2 out]
                n178 = property on="Test Slider" class="Slide (strict)"("Visible"=FALSE) -> ()  [unwired: 2 in, 2 out]
              }
              frame "White Balance  **" {
                n179 = Index Array(array=w309, index=1) -> (element=w310:cluster{string[]})
                n180 = call <vilib>:"NT Read String.vi"("Name"=w312) -> ("String"=w311:string)  [unwired: 9 in, 1 out]
                n181 = Unbundle(w310) -> (w307:string[])
                n182 = Match First String(2:w307, 3:w311) -> (0:w306:i32)  [unwired: 1 out]
                n183 = property on="Test Ring" class="Ring (strict)"("Value"=w306, "Strings []"=w307) -> ()  [unwired: 2 in, 2 out]
                n184 = property on="Test Ring" class="Ring (strict)"("Visible"=TRUE) -> ()  [unwired: 2 in, 2 out]
                n185 = property on="Test Slider" class="Slide (strict)"("Visible"=FALSE) -> ()  [unwired: 2 in, 2 out]
              }
              frame "Exposure  **" {
                n186 = Index Array(array=w318, index=2) -> (element=w319:cluster{string[]})
                n187 = call <vilib>:"NT Read String.vi"("Name"=w321) -> ("String"=w320:string)  [unwired: 9 in, 1 out]
                n188 = Unbundle(w319) -> (w315:string[])
                n189 = Match First String(2:w315, 3:w320) -> (0:w316:i32)  [unwired: 1 out]
                n190 = property on="Test Ring" class="Ring (strict)"("Value"=w316, "Strings []"=w315) -> ()  [unwired: 2 in, 2 out]
                n191 = property on="Test Ring" class="Ring (strict)"("Visible"=TRUE) -> ()  [unwired: 2 in, 2 out]
                n192 = property on="Test Slider" class="Slide (strict)"("Visible"=FALSE) -> ()  [unwired: 2 in, 2 out]
              }
              frame "Exposure Priority  **" {
                n193 = Index Array(array=w327, index=3) -> (element=w328:cluster{string[]})
                n194 = call <vilib>:"NT Read String.vi"("Name"=w330) -> ("String"=w329:string)  [unwired: 9 in, 1 out]
                n195 = Unbundle(w328) -> (w324:string[])
                n196 = Match First String(2:w324, 3:w329) -> (0:w325:i32)  [unwired: 1 out]
                n197 = property on="Test Ring" class="Ring (strict)"("Value"=w325, "Strings []"=w324) -> ()  [unwired: 2 in, 2 out]
                n198 = property on="Test Ring" class="Ring (strict)"("Visible"=TRUE) -> ()  [unwired: 2 in, 2 out]
                n199 = property on="Test Slider" class="Slide (strict)"("Visible"=FALSE) -> ()  [unwired: 2 in, 2 out]
              }
              frame "Color Enable  **" {
                n200 = Index Array(array=w336, index=4) -> (element=w337:cluster{string[]})
                n201 = call <vilib>:"NT Read String.vi"("Name"=w339) -> ("String"=w338:string)  [unwired: 9 in, 1 out]
                n202 = Unbundle(w337) -> (w333:string[])
                n203 = Match First String(2:w333, 3:w338) -> (0:w334:i32)  [unwired: 1 out]
                n204 = property on="Test Ring" class="Ring (strict)"("Value"=w334, "Strings []"=w333) -> ()  [unwired: 2 in, 2 out]
                n205 = property on="Test Ring" class="Ring (strict)"("Visible"=TRUE) -> ()  [unwired: 2 in, 2 out]
                n206 = property on="Test Slider" class="Slide (strict)"("Visible"=FALSE) -> ()  [unwired: 2 in, 2 out]
              }
              frame Default {
                n207 = property on="Test Ring" class="Ring (strict)"("Visible"=FALSE) -> ()  [unwired: 2 in, 2 out]
                n208 = property on="Test Slider" class="Slide (strict)"("Visible"=FALSE) -> ()  [unwired: 2 in, 2 out]
              }
              frame "Brightness  **", "Color Level  **", "Compression  **", "FPS  **", "Sharpness  **" {
                n209 = call <vilib>:"NT Read Number.vi"("Name"=w345) -> ("Numeric"=w344:dbl)  [unwired: 9 in, 1 out]
                n210 = local write "Test Slider"(w344) -> ()
                n211 = property on="Test Slider" class="Slide (strict)"("Visible"=TRUE, "Scale.Maximum"=100.0 ("Scale.Range:Maximum")) -> ()  [unwired: 2 in, 2 out]
                n212 = property on="Test Ring" class="Ring (strict)"("Visible"=FALSE) -> ()  [unwired: 2 in, 2 out]
              }
            }
          }
        }
        n213 = property on="Progress" class="Clust (strict)"("Visible"=FALSE) -> ()  [unwired: 2 in, 2 out]
      }
      event "Test Name": Mouse Enter {
        # "Populate the ring with the list of tests"
        n214 = event-data() -> ()  [unwired: 1 in, 1 out]
        n215 = call <vilib>:"NT Read String Array.vi"("Name"="TestMode/TestList") -> ("String Array"=w353:string[])  [unwired: 9 in, 1 out]
        n216 = Build Array (concatenate)("Select the test to run...", w353) -> (w352:string[])
        n217 = property on="Test Name" class="Ring (strict)"("Strings []"=w352) -> ()  [unwired: 2 in, 2 out]
      }
      event "Test Name": Value Change {
        w355 = FALSE ("Visible")
        # "Tell the robot the test name to run"
        n218 = event-data() -> ("NewVal"=w359:u16)  [unwired: 1 in]
        n219 = property on="Test Name" class="Ring (strict)"() -> ("Strings []"=w360:string[])  [unwired: 2 in, 2 out]
        n220 = local write "Progress"(T8 {"Test Progress"=0, "Test Progress Text"=""} ("Progress")) -> ()
        n221 = Index Array(array=w360, index=w359) -> (element=w358:string)
        n222 = call <vilib>:"NT Write String.vi"("String"=w358, "Name"="TestMode/TestName") -> ()  [unwired: 9 in, 1 out]
        n223 = property on="Progress" class="Clust (strict)"("Visible"=TRUE) -> ()  [unwired: 2 in, 2 out]
        n224 = property on="Motor" class="Clust (strict)"("Visible"=w355) -> ()  [unwired: 2 in, 2 out]
        n225 = property on="Test Slider" class="Slide (strict)"("Visible"=w355) -> ()  [unwired: 2 in, 2 out]
        n226 = property on="On/Off" class="Bool (strict)"("Visible"=w355) -> ()  [unwired: 2 in, 2 out]
        n227 = property on="Rev/Fwd" class="Clust (strict)"("Visible"=w355) -> ()  [unwired: 2 in, 2 out]
        n228 = property on="Test Ring" class="Ring (strict)"("Visible"=w355) -> ()  [unwired: 2 in, 2 out]
      }
      event "Select Auto": Mouse Enter {
        # "Populate the combo box with the list of autonomous options"
        n229 = event-data() -> ()  [unwired: 1 in, 1 out]
        n230 = call <vilib>:"NT Read String Array.vi"("Name"="Auto List") -> ("String Array"=w362:string[])  [unwired: 9 in, 1 out]
        n231 = property on="Select Auto" class="CmbBox"("Strings[]"=w362) -> ()  [unwired: 2 in, 2 out]
      }
      event "Select Auto": Value Change {
        # "User modified the Auto Selection. Write to NT variable so robot knows."
        n232 = event-data() -> ("NewVal"=w365:string)  [unwired: 1 in]
        n233 = call <vilib>:"NT Write String.vi"("String"=w365, "Name"="Auto Selector") -> ()  [unwired: 9 in, 1 out]
      }
      event "Command Selection": Value Change {
        # "Get the params and show in table"
        n234 = event-data() -> ("NewVal"=w371:i32)  [unwired: 1 in]
        n235 = property on="Command Selection" class="MCListbox (strict)"() -> ("ItemNames"=w369:string[][])  [unwired: 2 in, 2 out]
        n236 = call <vilib>:"WPI_DashboardUpdate Command Params.vi"("NewVal"=w371, "Commands"=w369, "Param Tbl"=w370) -> ()  [unwired: 8 in, 1 out]
      }
      event "Execute Command": Value Change {
        # "Started one, Unique ID holds\nresponse"
        n237 = event-data() -> ()  [unwired: 1 in, 1 out]
        n238 = property on="Command Selection" class="MCListbox (strict)"() -> ("ItemNames"=w382:string[][])  [unwired: 2 in, 2 out]
        n239 = Index Array(array=w382, index (row)="Command Selection", index (col)=0) -> (element=w380:string)
        n240 = call <vilib>:"Invoke Commands.vi"("Command Params"="Command Params", "Function Name"=w380) -> ("Params"=w376:u8, "Started"=w375:bool)  [unwired: 7 in, 1 out]
        n241 = Array Subset(array="Command Params", length (row)=w376) -> (w377:string[][])  [unwired: 3 in]
        n242 = Select(t="Executing" ("Cmd Status"), s=w375, f="" ("Cmd Status")) -> (s? t:f=→"Cmd Status":string)
      }
      event "Command Selection": Double Click {
        n243 = event-data() -> ("Row"=w390:i32)  [unwired: 1 in]
        n244 = property on="Command Selection" class="MCListbox (strict)"() -> ("ItemNames"=w393:string[][])  [unwired: 2 in, 2 out]
        n245 = local read "Command Params"() -> (w389:string[][])
        n246 = Index Array(array=w393, index (row)=w390, index (col)=0) -> (element=w391:string)
        n247 = call <vilib>:"Invoke Commands.vi"("Command Params"=w389, "Function Name"=w391) -> ("Params"=w388:u8, "Started"=w383:bool)  [unwired: 7 in, 1 out]
        n248 = Array Subset(array=w389, length (row)=w388) -> (w387:string[][])  [unwired: 3 in]
        n249 = Select(t="Executing" ("Cmd Status"), s=w383, f="" ("Cmd Status")) -> (s? t:f=w384:string)
        n250 = local write "Cmd Status"(w384) -> ()
      }
      event "CheckList": Double Click {
        # "Shift clears all"
        # "Update symbols on the listbox"
        n251 = event-data() -> ("PlatMods.Shift"=w395:bool, "Row"=w397:i32)  [unwired: 1 in]
        n252 = case shown="True" w395 {
          tunnel: w397 -> [w401 _]
          tunnel: 1 -> [w400 _]
          frame False {
            n253 = property on="CheckList" class="LstBox (strict)"() -> ("Item Symbols"=w399:i32[])  [unwired: 2 in, 2 out]
            n254 = Replace Array Subset(array=w399, new element=w400, index=w401) -> (w398:i32[])
            n255 = property on="CheckList" class="LstBox (strict)"("Item Symbols"=w398) -> ()  [unwired: 2 in, 2 out]
          }
          frame True {
            w402 = 0 ("Top Row")
            n256 = property on="CheckList" class="LstBox (strict)"() -> ("Number of Rows"=w404:u32)  [unwired: 2 in, 2 out]
            n257 = Initialize Array(0, w404) -> (w403:i32[])
            n258 = property on="CheckList" class="LstBox (strict)"("Top Row"=w402, "Value"=w402, "Item Symbols"=w403) -> ()  [unwired: 2 in, 2 out]
          }
        }
      }
      event "CheckList": Key Down {
        # "Update symbols on the listbox\nLeft and right keys check and uncheck"
        n259 = event-data() -> ("VKey"=w408:T25)  [unwired: 1 in]
        n260 = case shown="\"Left\", \"Right\"" w408 {
          selector: w408 -> [w413 _]
          tunnel: eventvkey."Left" ("VKey") -> [w411 _]
          frame "Left", "Right" {
            n261 = Equal?(x=w411, y=w413) -> (x = y?=w412:bool)
            n262 = Select(t=0, s=w412, f=1) -> (s? t:f=w414:i32)
            n263 = property on="CheckList" class="LstBox (strict)"() -> ("Item Symbols"=w417:i32[])  [unwired: 2 in, 2 out]
            n264 = Replace Array Subset(array=w417, new element=w414, index="CheckList") -> (w416:i32[])
            n265 = property on="CheckList" class="LstBox (strict)"("Item Symbols"=w416) -> ()  [unwired: 2 in, 2 out]
          }
          frame Default {
          }
        }
      }
      event "Motor.Enable": Value Change {
        # "When the test mode otor enable helper is set, update that\ntree row item's value"
        n266 = event-data() -> ("NewVal"=w423:bool)  [unwired: 1 in]
        n267 = Unbundle("Motor") -> ("Value"=w422:dbl)  [unwired: 1 out]
        n268 = Select(t=w422, s=w423, f=0.0) -> (s? t:f=w420:dbl)
        n269 = call <vilib>:"NT Write Number.vi"("Numeric"=w420, "Name"=w419) -> ()  [unwired: 9 in, 1 out]
      }
      event "Test Slider": Value Change {
        # "When the test mode slider helper is set, update that\ntree row item's value"
        n270 = event-data() -> ("NewVal"=w426:dbl)  [unwired: 1 in]
        n271 = call <vilib>:"NT Write Number.vi"("Numeric"=w426, "Name"=w427) -> ()  [unwired: 9 in, 1 out]
      }
      event "On/Off": Value Change {
        # "When the test mode on/off helper value is set, update that\ntree row item's value"
        n272 = event-data() -> ("NewVal"=w431:bool)  [unwired: 1 in]
        n273 = Boolean To (0,1)(Boolean=w431) -> (0, 1=w430:i16)
        n274 = call <vilib>:"NT Write Number.vi"("Numeric"=w430, "Name"=w429) -> ()  [unwired: 9 in, 1 out]
      }
      event "Rev/Fwd": Value Change {
        # "When the test mode helper value for relays is set, update that\ntree row item's value"
        n275 = event-data() -> ("NewVal.Forward"=w439:bool, "NewVal.Reverse"=w438:bool)  [unwired: 1 in]
        n276 = Boolean To (0,1)(Boolean=w439) -> (0, 1=w435:i16)
        n277 = Boolean To (0,1)(Boolean=w438) -> (0, 1=w437:i16)
        n278 = Negate(x=w437) -> (-x=w436:i16)
        n279 = Add(x=w435, y=w436) -> (x+y=w434:i16)
        n280 = call <vilib>:"NT Write Number.vi"("Numeric"=w434, "Name"=w433) -> ()  [unwired: 9 in, 1 out]
      }
      event "Test Ring": Value Change {
        # "When a test mode helper value is selected from the ring,\nset the tree item's variable to the string value"
        n281 = event-data() -> ("NewVal"=w443:u16)  [unwired: 1 in]
        n282 = property on="Test Ring" class="Ring (strict)"() -> ("Strings []"=w444:string[])  [unwired: 2 in, 2 out]
        n283 = Index Array(array=w444, index=w443) -> (element=w442:string)
        n284 = call <vilib>:"NT Write String.vi"("String"=w442, "Name"=w441) -> ()  [unwired: 9 in, 1 out]
      }
      event "Rec Mode": Value Change {
        # "Update globals for recording mode and path to read log from.\nClear when logging and let NetworkTables set path for vision to\nuse."
        n285 = event-data() -> ("NewVal"=w455:enum32{"Stop", "Record", "Playback"})  [unwired: 1 in]
        n286 = global write "WPI_DashboardLogging Global.vi" "Logging Filename"(path "") -> ()
        n287 = global write "WPI_DashboardLogging Global.vi" "Recording"(w455) -> ()
        n288 = case shown="\"Playback\"" w455 {
          tunnel: w454 -> [_ w457 w466]
          tunnel: [_ _ w465] -> w452
          tunnel: [_ _ w464] -> _
          tunnel: w450 -> [_ _ w462]
          tunnel: cluster{i32, i32} {-250, 170} -> [_ _ w461]
          tunnel: [_ _ T26 {"Image Size"=TRUE, "Image Type"=TRUE, "Pixel Value"=TRUE, "ROI Information"=TRUE, "Zoom Factor"=FALSE} ("Image Information Shown:All Elements")] -> w445
          tunnel: [_ _ TRUE ("Zoom Factor")] -> w446
          tunnel: w448 -> [_ _ w458]
          frame Default {
          }
          frame "Stop", "Record" {
            # "Place Window too"
            n289 = invoke class="VI" method="FP.Close"(reference=w457) -> (reference out=w456:refnum<vi>)  [unwired: 2 in, 2 out]
            n290 = invoke class="VI" method="Abort VI"(reference=w456) -> ()  [unwired: 2 in, 3 out]
          }
          frame "Playback" {
            n291 = call "Open Playback Panel.vi"("Offset"=w461, "DB VI Ref"=w462, "Playback in"=w466) -> ("Playback out"=w463:refnum<vi>)  [unwired: 8 in]
            n292 = register-events(w463, w458) -> (reference out=w465:refnum<event-registration>, error out=w464:errorcluster)  [unwired: 2 in]
          }
        }
        n293 = property on="Camera Image Right" class="ImageControl"("Image Information Shown"=w445, "Image Information Visible"=w446) -> ()  [unwired: 2 in, 2 out]
        n294 = property on="Camera Image" class="ImageControl"("Image Information Shown"=w445, "Image Information Visible"=w446) -> ()  [unwired: 2 in, 2 out]
        n295 = call <vilib>:"WPI_DashboardNT Log FieldName Cache.vi"("Operation"=enum16{"Lookup/Add", "Index", "Clear"}."Clear") -> ()  [unwired: 8 in, 3 out]
      }
      event Panel Close {
        w468 = enum32{"Stop", "Record", "Playback"}."Stop" ("Rec Mode")
        # "Playback window has been closed, abort"
        n296 = event-data() -> ()  [unwired: 1 in, 4 out]
        n297 = local write "Rec Mode"(w468) -> ()
        n298 = global write "WPI_DashboardLogging Global.vi" "Recording"(w468) -> ()
      }
      event Panel Close {
        # "Abort playback window and ourself"
        n299 = event-data() -> ()  [unwired: 1 in, 4 out]
        n300 = invoke class="VI" method="FP.Close"(reference=w472) -> (reference out=w471:refnum<vi>)  [unwired: 2 in, 2 out]
        n301 = invoke class="VI" method="Abort VI"(reference=w471) -> (error out=w470:errorcluster)  [unwired: 2 in, 2 out]
        n302 = invoke class="VI" method="Abort VI"(error in=w470) -> ()  [unwired: 2 in, 3 out]
      }
      event User Event {
        n303 = event-data() -> ("IDs"=w479:cluster{"RPC field ID":u16, "Unique ID":u16}, "String"=w478:string)  [unwired: 1 in]
        n304 = Bundle("IDs"=w479, "String"=w478) -> (w477:T11)  [unwired: 1 in]
        n305 = call <vilib>:"Retrieve RPC Response.vi"("RPC Response"=w477) -> ("Output"=w475:string[][])  [unwired: 10 in]
        n306 = Build Array (concatenate)(w473, w475) -> (w474:string[][])
        n307 = local write "Command Params"(w474) -> ()
        n308 = local write "Cmd Status"("" ("Cmd Status")) -> ()
      }
      event "Tree": Double Click {
        n309 = event-data() -> ("PlatMods"=w485:T29, "Tag"=w482:string)  [unwired: 1 in]
        n310 = Unbundle(w485) -> ("Shift"=w484:bool)  [unwired: 4 out]
        n311 = String Subset(string=w482, length (rest)=1 ("length (rest)")) -> (substring=w481:string)  [unwired: 1 in]
        n312 = Not(x=w484) -> (.not. x?=w483:bool)
        n313 = case shown="\"/\"" w481 {
          tunnel: w482 -> [_ w488]
          tunnel: w483 -> [_ w487]
          frame Default {
          }
          frame "/" {
            n314 = call <vilib>:"NT Update Persistence.vi"("Persistence"=w487, "Name"=w488) -> ()  [unwired: 9 in, 1 out]
          }
        }
      }
    }
  }
  n315 = while {
    tunnel: w65 -> [w490]
    i -> [w493]
    stop <- FALSE stop-if-true
    n316 = Wait (ms)(milliseconds to wait=u32 100) -> ()  [unwired: 1 out]
    n317 = case shown="\"Playback\"" "Rec Mode" {
      tunnel: w493 -> [_ _ w508]
      tunnel: [u32 2829099 ("Base Color") u32 11141120 ("Target Color") w497] -> w489
      frame "Stop", Default {
        # "Reset the color, extra updates don't cost much"
      }
      frame "Record" {
      }
      frame "Playback" {
        # "Playback"
        n318 = Quotient & Remainder(x=w508, y=u32 50 ("milliseconds to wait")) -> (x-y*floor(x/y)=w504:u32)  [unwired: 1 out]
        n319 = Divide(x=w504, y=u32 50 ("milliseconds to wait")) -> (x/y=w501:dbl)
        n320 = Multiply(x=6.283185307179586, y=w501) -> (x*y=w506:dbl)
        n321 = Sine(x=w506) -> (sin(x)=w505:dbl)
        n322 = Absolute Value(x=w505) -> (abs(x)=w498:dbl)
        n323 = call "Interpolate RGB Color.vi"("Proportion"=w498, "Target Color"=u32 30976, "Base Color"=u32 2829099) -> ("Result Color"=w497:u32)  [unwired: 8 in]
      }
    }
    n324 = property class="Pane"(reference=w490, "PaneColor"=w489) -> ()  [unwired: 1 in, 2 out]
  }
  n325 = local write "Dashboard Tab"(T2."Drive" ("Dashboard Tab")) -> ()
  n326 = property on="On/Off" class="Bool (strict)"("Visible"=w36) -> ()  [unwired: 2 in, 2 out]
  n327 = property on="Motor" class="Clust (strict)"("Visible"=w36) -> ()  [unwired: 2 in, 2 out]
  n328 = property on="Progress" class="Clust (strict)"("Visible"=w36) -> ()  [unwired: 2 in, 2 out]
  n329 = property on="Test Ring" class="Ring (strict)"("Visible"=w36) -> ()  [unwired: 2 in, 2 out]
  n330 = property on="Rev/Fwd" class="Clust (strict)"("Visible"=w36) -> ()  [unwired: 2 in, 2 out]
  n331 = while {
    tunnel: u16 1741 ("timeout ms (25000)") -> [w510]
    stop <- FALSE stop-if-true
    n332 = TCP Create Listener(10:w510) -> (0:w509:errorcluster, 3:w511:refnum<k5>)  [unwired: 4 in, 1 out]
    n333 = case shown="No Error" w509 {
      selector: w509 -> [w513 _]
      tunnel: w511 -> [w514 _]
      frame No Error {
        n334 = while {
          tunnel: w514 -> [w517]
          tunnel: w513 -> [w516]
          stop <- FALSE stop-if-true
          n335 = TCP Wait On Listener(8:w516, 11:w517) -> (0:w518:errorcluster, 4:w519:refnum<k5>)  [unwired: 2 in, 3 out]
          n336 = local write "TCP"(w519) -> ()
          n337 = case shown="No Error" w518 {
            frame No Error {
            }
            frame Error {
              n338 = Wait (ms)(milliseconds to wait=u32 1000) -> ()  [unwired: 1 out]
            }
          }
        }
      }
      frame Error {
        n339 = Wait (ms)(milliseconds to wait=u32 1000) -> ()  [unwired: 1 out]
      }
    }
  }
  n340 = local write "Command Selection"(u16 0 ("milliseconds to wait")) -> ()
  n341 = local write "Command Params"(string[][] [] ("Command Params")) -> ()
  n342 = global write "WPI_DashboardLogging Global.vi" "Recording"(w59) -> ()
  n343 = local write "Rec Mode"(w59) -> ()
  n344 = call <vilib>:"NT Write String.vi"("String"="Select Auto", "Name"="Auto Selector") -> ()  [unwired: 9 in, 1 out]
